vi "Element Init.vi"(7 "VolatusAPI":refnum<class "VolatusAPI.lvclass">, 8 "error in (no error)":errorcluster, 10 "JSON":string, 11 "ButtonControl in":refnum<class "DigitalButtonControl.lvclass">) -> (0 "error out":errorcluster, 3 "ButtonControl out":refnum<class "DigitalButtonControl.lvclass">)   [LabVIEW 2020, in "VolatusGUIElements.lvlib" / "DigitalButtonControl.lvclass"]
uses:
  DigitalButtonControl.lvclass
  C:/dev/lv20CE/relink/lv-volatus/VolatusGUI/GUI Element/GUI Element.lvclass
  Volatus/VolatusAPI/VolatusAPI.lvclass
  lv-vecto/Vecto/Group DBL/Group DBL.lvclass
  C:/dev/lv20CE/relink/lv-vecto/Vecto/Group/Group.lvclass
  VolatusGUI/GUI Element/GUI Element.lvclass/GUI Element.ctl
  DigitalButtonControl.lvclass/DigitalButtonControl.ctl
  7f1ddf9b-cd10-40fa-bddf-b675369dd94f.vi
  <vilib>/JDP Science/JSONtext/JSON text to Variant.vi
  <vilib>/JDP Science/JSONtext/LVClass Serializer/JSONtext LVClass Serializer.lvclass
  VolatusGUI/GUI Element/GUI Element.lvclass
  VolatusGUI/Element Inhibit/Element Inhibit.lvclass
  Volatus/Digital Command/Digital Command.lvclass
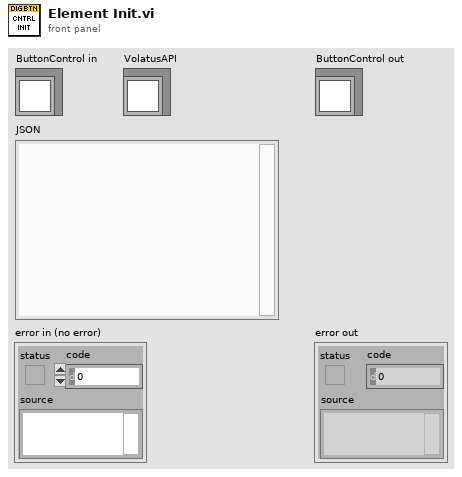
[diagram p1: front panel]
types:
  T1 = typedef "VolatusGUIElements.lvlib/DigitalButtonControl.lvclass/JSON.ctl" = cluster{"Channel":string, "Staleness":dbl, "Inhibit":string}
  T2 = typedef "VectoConfig.lvlib/Channel Info.ctl" = cluster{"Name":string, "Group":string, "Owning Node":string, "Owning Task":string, "Resource":string}
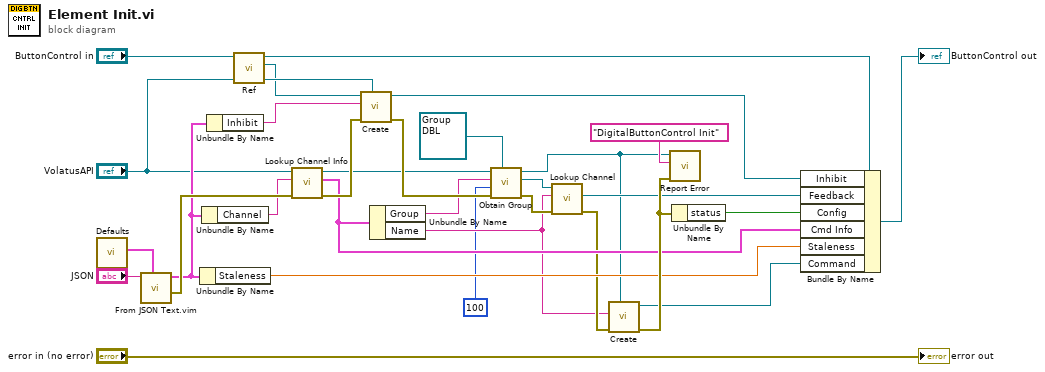
[diagram p0: block diagram]
diagram:
  n1 = call "Defaults.vi"() -> ("Defaults"=w19:T1)  [unwired: 11 in]
  n2 = call "From JSON Text.vim"("Data Type and Default Value"=w19, "JSON"="JSON") -> ("error out"=w28:errorcluster, "Data out"=w11:T1)  [unwired: 8 in]
  n3 = Unbundle By Name(w11) -> ("Staleness"=w17:dbl)
  n4 = Unbundle By Name(w11) -> ("Channel"=w15:string)
  n5 = Unbundle By Name(w11) -> ("Inhibit"=w10:string)
  n6 = call "Ref.vi"("GUI Element in"="ButtonControl in") -> ("Ref"=w8:refnum<vi>, "GUI Element out"=w25:refnum<class "DigitalButtonControl.lvclass">)  [unwired: 9 in]
  n7 = call "Lookup Channel Info.vi"("error in (no error)"=w28, "Channel Name"=w15, "VolatusAPI in"="VolatusAPI") -> ("error out"=w29:errorcluster, "Channel Info"=w13:T2, "VolatusAPI out"=w16:refnum<class "VolatusAPI.lvclass">)  [unwired: 5 in, 1 out]
  n8 = call "Create.vi"("VolatusAPI"="VolatusAPI", "error in (no error)"=w29, "Inhibit Channel"=w10, "Control Ref"=w8) -> ("error out"=w30:errorcluster, "Element Inhibit out"=w7:refnum<class "Element Inhibit.lvclass">)  [unwired: 6 in]
  n9 = Unbundle By Name(w13) -> ("Group"=w14:string, "Name"=w4:string)
  n10 = call "Obtain Group.vi"("Group Type (Abstract)"=refnum<class "Group DBL.lvclass"> refnum ("Vecto.lvlib:Group.lvclass"), "error in (no error)"=w30, "Timeout ms (5000)"=u32 100, "Group Name"=w14, "VolatusAPI in"=w16) -> ("error out"=w22:errorcluster, "Group"=w23:refnum<class "Group DBL.lvclass">, "VolatusAPI out"=w3:refnum<class "VolatusAPI.lvclass">)  [unwired: 4 in]
  n11 = call "Lookup Channel.vi"("error in (no error)"=w22, "Channel Name"=w4, "Group in"=w23) -> ("error out"=w5:errorcluster, "Channel"=w20:refnum<class "Channel DBL.lvclass">)  [unwired: 6 in, 1 out]
  n12 = call "Create.vi"("VolatusAPI"=w3, "error in (no error)"=w5, "Channel"=w4) -> ("error out"=w31:errorcluster, "Digital Command out"=w2:refnum<class "Digital Command.lvclass">)  [unwired: 7 in]
  n13 = call "Report Error.vi"("error in (no error)"=w31, "Context"="DigitalButtonControl Init", "VolatusAPI in"=w3) -> ()  [unwired: 7 in, 2 out]
  n14 = Unbundle By Name(w31) -> ("status"=w12:bool)
  n15 = Bundle By Name(cluster=w25, "Inhibit"=w7, "Feedback"=w20, "Config"=w12, "Cmd Info"=w13, "Staleness"=w17, "Command"=w2) -> (→"ButtonControl out":refnum<class "DigitalButtonControl.lvclass">)
  "error out" <- "error in (no error)"
